vi "EOL Check Sunshade Limits.vi"(7 "Pass? In":bool=TRUE, 8 "Error Table":string[][](array[string]), 9 "Sunshade Close?":bool=TRUE, 10 "Sun Shade Limits":T1 {"Variance" format="%.2g"; "Truncation End" format="%.2g"; "Truncation Start" format="%.2g"; "Avg Max" format="%.2g"; "Avg Min" format="%.2g"; "Overall Max" format="%.2g"; "Overall Min" format="%.2g"}, 11 "Sunshade Calculated Data":dbl[](array[numeric])) -> (0 "Error Table 2":string[][](array[string]), 2 "All Sunshade Data and Limits":dbl[](array[numeric]), 3 "Pass?":bool)   [LabVIEW 2018]
uses:
  05.UserVI's/type defs/17x Sunshade Limts Seq.ctl
panel:
  # "Min"
  # "N"
  # "Min"
  # "Start"
  # "N"
  # "Max"
  # "N"
  # "Max"
  # "N"
  # "End"
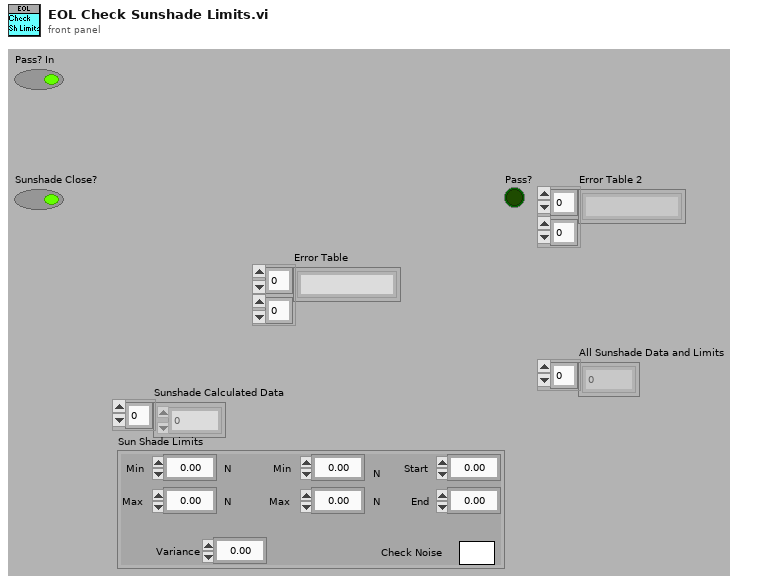
[diagram p1: front panel]
types:
  T1 = typedef "17x Sunshade Limts Seq.ctl" = cluster{"Overall Min":dbl, "Overall Max":dbl, "Avg Min":dbl, "Avg Max":dbl, "Truncation Start":dbl, "Truncation End":dbl, "Variance":dbl, "Check Noise":bool}
  T2 = cluster{"Sunshade Calculated Data":dbl[], "Sun Shade Limits":T1, "Error Table":string[][], "Sunshade Close?":bool, "Pass? In":bool}
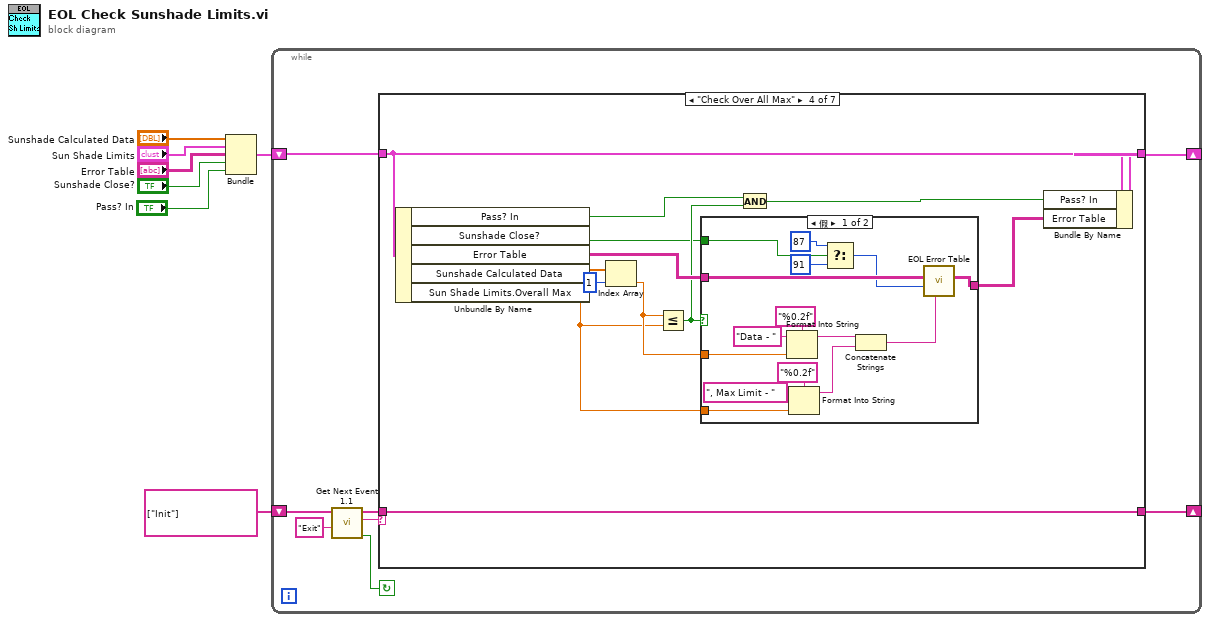
[diagram p0: block diagram]
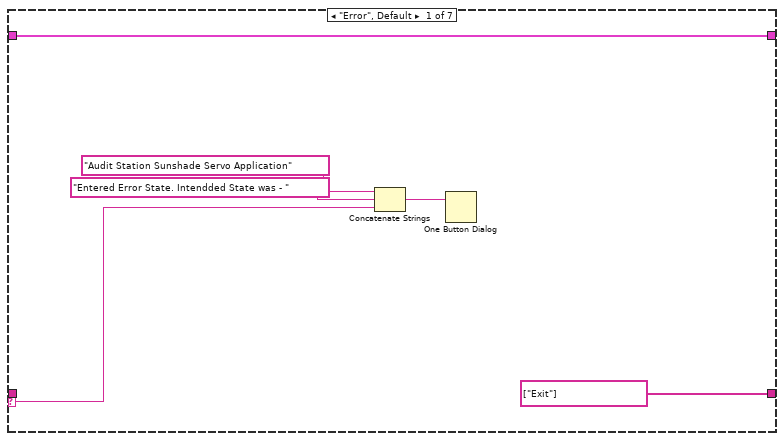
[diagram p2: hidden frame]
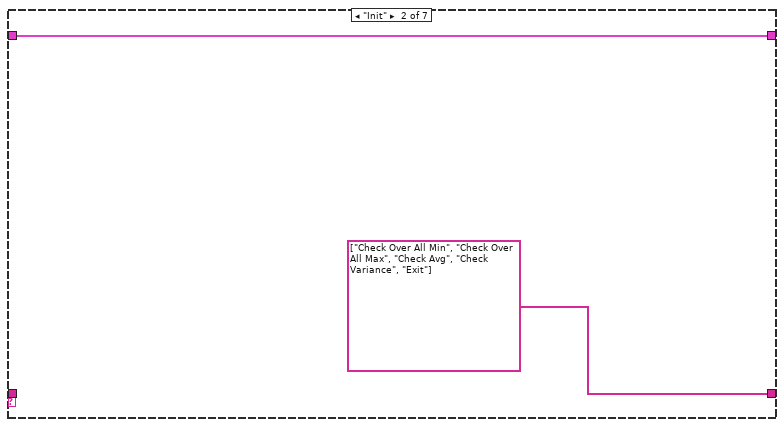
[diagram p3: hidden frame]
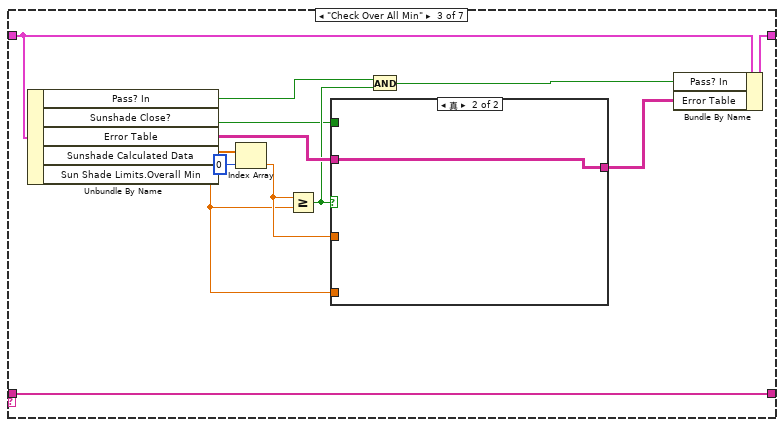
[diagram p4: hidden frame]
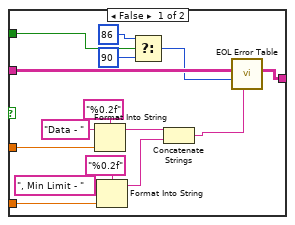
[diagram p5: hidden frame]
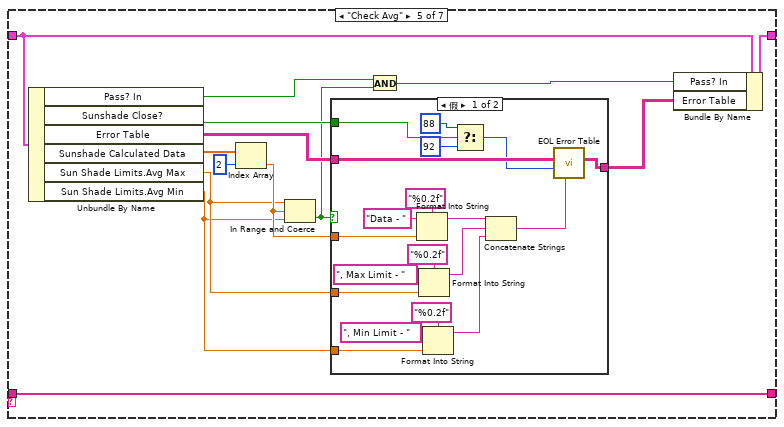
[diagram p7: hidden frame]
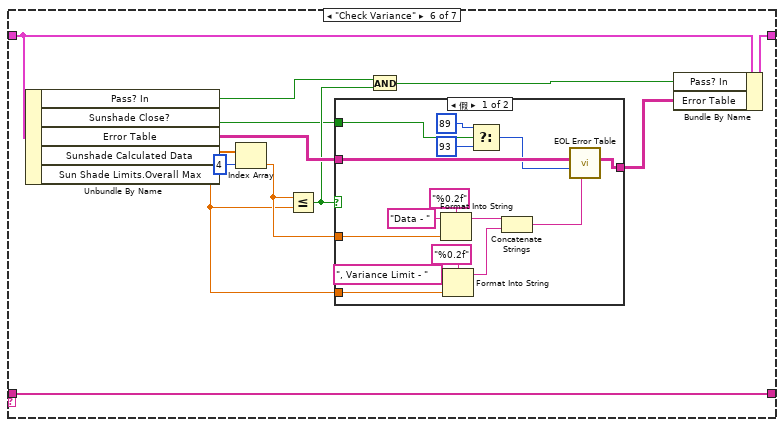
[diagram p9: hidden frame]
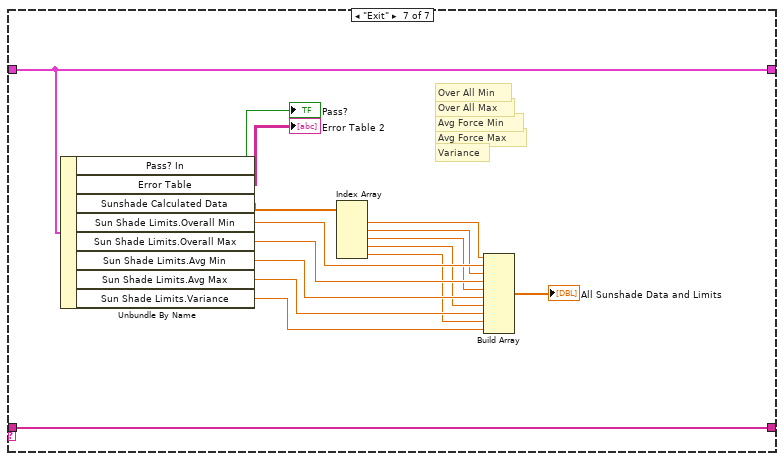
[diagram p11: hidden frame]
diagram:
  n1 = Bundle("Sunshade Calculated Data"="Sunshade Calculated Data", "Sun Shade Limits"="Sun Shade Limits", "Error Table"="Error Table", "Sunshade Close?"="Sunshade Close?", "Pass? In"="Pass? In") -> (w2:T2)  [unwired: 1 in]
  n2 = while {
    shift-right: [w11] -> _
    shift-left: string[] ["Init"] ("event queue out") -> [w10]
    shift-right: [w8] -> _
    shift-left: w2 -> [w9]
    stop <- w14 continue-if-true
    n3 = call "Get Next Event 1.1.vi"("Exit Event"="Exit", "event queue in"=w10) -> ("Condition (Exit:F)"=w14:bool, "next event"=w15:string, "event queue out"=w12:string[])  [unwired: 6 in, 1 out]
    n4 = case shown="\"Check Over All Max\"" w15 {
      selector: w15 -> [w17 _ _ _ _ _ _]
      tunnel: w12 -> [_ _ w29 w58 w89 w121 w160]
      tunnel: [string[] ["Exit"] ("event queue out") string[] ["Check Over All Min", "Check Over All Max", "Check Avg", "Check Variance", "Exit"] ("event queue out") w29 w58 w89 w121 w160] -> w11
      tunnel: w9 -> [w16 w23 w34 w63 w93 w126 w159]
      tunnel: [w16 w23 w30 w59 w90 w122 w159] -> w8
      frame "Error", Default {
        n5 = Concatenate Strings("Audit Station Sunshade Servo Application" ("string"), "Entered Error State. Intendded State was - " ("string"), w17) -> (w20:string)
        n6 = One Button Dialog(message=w20) -> ()  [unwired: 1 in, 1 out]
      }
      frame "Init" {
      }
      frame "Check Over All Min" {
        n7 = Unbundle By Name(w34) -> ("Pass? In"=w33:bool, "Sunshade Close?"=w25:bool, "Error Table"=w35:string[][], "Sunshade Calculated Data"=w36:dbl[], "Sun Shade Limits.Overall Min"=w26:dbl)
        n8 = Index Array(array=w36, index=0) -> (element=w27:dbl)
        n9 = Greater Or Equal?(x=w27, y=w26) -> (x >= y?=w32:bool)
        n10 = case shown="真" w32 {
          tunnel: w35 -> [w51 w52]
          tunnel: w26 -> [w48 _]
          tunnel: [w37 w52] -> w28
          tunnel: w27 -> [w43 _]
          tunnel: w25 -> [w42 _]
          frame False {
            n11 = Format Into String(format string="%0.2f", initial string="Data - ", w43) -> (resulting string=w45:string)  [unwired: 1 in, 1 out]
            n12 = Format Into String(format string="%0.2f", initial string=", Min Limit - ", w48) -> (resulting string=w44:string)  [unwired: 1 in, 1 out]
            n13 = Select(t=u16 86 ("Error No."), s=w42, f=u16 90) -> (s? t:f=w38:u16)
            n14 = Concatenate Strings(w45, w44) -> (w39:string)
            n15 = call "EOL Error Table.vi"("Error Description"=w39, "Error No."=w38, "Error Table In"=w51) -> ("Error Table Out"=w37:string[][])  [unwired: 7 in, 1 out]
          }
          frame True {
          }
        }
        n16 = And(x=w33, y=w32) -> (x .and. y?=w31:bool)
        n17 = Bundle By Name(cluster=w34, "Pass? In"=w31, "Error Table"=w28) -> (w30:T2)
      }
      frame "Check Over All Max" {
        n18 = Unbundle By Name(w63) -> ("Pass? In"=w62:bool, "Sunshade Close?"=w54:bool, "Error Table"=w64:string[][], "Sunshade Calculated Data"=w65:dbl[], "Sun Shade Limits.Overall Max"=w55:dbl)
        n19 = Index Array(array=w65, index=1) -> (element=w56:dbl)
        n20 = Less Or Equal?(x=w56, y=w55) -> (x <= y?=w61:bool)
        n21 = case shown="假" w61 {
          tunnel: w64 -> [w80 w81]
          tunnel: w55 -> [w77 _]
          tunnel: [w66 w81] -> w57
          tunnel: w56 -> [w72 _]
          tunnel: w54 -> [w71 _]
          frame False {
            n22 = Format Into String(format string="%0.2f", initial string="Data - ", w72) -> (resulting string=w74:string)  [unwired: 1 in, 1 out]
            n23 = Format Into String(format string="%0.2f", initial string=", Max Limit - ", w77) -> (resulting string=w73:string)  [unwired: 1 in, 1 out]
            n24 = Select(t=u16 87 ("Error No."), s=w71, f=u16 91) -> (s? t:f=w67:u16)
            n25 = Concatenate Strings(w74, w73) -> (w68:string)
            n26 = call "EOL Error Table.vi"("Error Description"=w68, "Error No."=w67, "Error Table In"=w80) -> ("Error Table Out"=w66:string[][])  [unwired: 7 in, 1 out]
          }
          frame True {
          }
        }
        n27 = And(x=w62, y=w61) -> (x .and. y?=w60:bool)
        n28 = Bundle By Name(cluster=w63, "Pass? In"=w60, "Error Table"=w57) -> (w59:T2)
      }
      frame "Check Avg" {
        n29 = Unbundle By Name(w93) -> ("Pass? In"=w92:bool, "Sunshade Close?"=w87:bool, "Error Table"=w94:string[][], "Sunshade Calculated Data"=w95:dbl[], "Sun Shade Limits.Avg Max"=w84:dbl, "Sun Shade Limits.Avg Min"=w82:dbl)
        n30 = Index Array(array=w95, index=2) -> (element=w85:dbl)
        n31 = In Range and Coerce(upper limit=w84, x=w85, lower limit=w82) -> (In Range?=w83:bool)  [unwired: 1 out]
        n32 = case shown="假" w83 {
          tunnel: w94 -> [w114 w115]
          tunnel: w84 -> [w111 _]
          tunnel: [w96 w115] -> w88
          tunnel: w85 -> [w106 _]
          tunnel: w87 -> [w105 _]
          tunnel: w82 -> [w100 _]
          frame False {
            n33 = Format Into String(format string="%0.2f", initial string="Data - ", w106) -> (resulting string=w108:string)  [unwired: 1 in, 1 out]
            n34 = Format Into String(format string="%0.2f", initial string=", Max Limit - ", w111) -> (resulting string=w107:string)  [unwired: 1 in, 1 out]
            n35 = Format Into String(format string="%0.2f", initial string=", Min Limit - ", w100) -> (resulting string=w99:string)  [unwired: 1 in, 1 out]
            n36 = Select(t=u16 88 ("Error No."), s=w105, f=u16 92) -> (s? t:f=w97:u16)
            n37 = Concatenate Strings(w108, w107, w99) -> (w98:string)
            n38 = call "EOL Error Table.vi"("Error Description"=w98, "Error No."=w97, "Error Table In"=w114) -> ("Error Table Out"=w96:string[][])  [unwired: 7 in, 1 out]
          }
          frame True {
          }
        }
        n39 = And(x=w92, y=w83) -> (x .and. y?=w91:bool)
        n40 = Bundle By Name(cluster=w93, "Pass? In"=w91, "Error Table"=w88) -> (w90:T2)
      }
      frame "Check Variance" {
        n41 = Unbundle By Name(w126) -> ("Pass? In"=w125:bool, "Sunshade Close?"=w117:bool, "Error Table"=w127:string[][], "Sunshade Calculated Data"=w128:dbl[], "Sun Shade Limits.Overall Max"=w118:dbl)
        n42 = Index Array(array=w128, index=4) -> (element=w119:dbl)
        n43 = Less Or Equal?(x=w119, y=w118) -> (x <= y?=w124:bool)
        n44 = case shown="假" w124 {
          tunnel: w127 -> [w143 w144]
          tunnel: w118 -> [w140 _]
          tunnel: [w129 w144] -> w120
          tunnel: w119 -> [w135 _]
          tunnel: w117 -> [w134 _]
          frame False {
            n45 = Format Into String(format string="%0.2f", initial string="Data - ", w135) -> (resulting string=w137:string)  [unwired: 1 in, 1 out]
            n46 = Format Into String(format string="%0.2f", initial string=", Variance Limit - ", w140) -> (resulting string=w136:string)  [unwired: 1 in, 1 out]
            n47 = Select(t=u16 89 ("Error No."), s=w134, f=u16 93) -> (s? t:f=w130:u16)
            n48 = Concatenate Strings(w137, w136) -> (w131:string)
            n49 = call "EOL Error Table.vi"("Error Description"=w131, "Error No."=w130, "Error Table In"=w143) -> ("Error Table Out"=w129:string[][])  [unwired: 7 in, 1 out]
          }
          frame True {
          }
        }
        n50 = And(x=w125, y=w124) -> (x .and. y?=w123:bool)
        n51 = Bundle By Name(cluster=w126, "Pass? In"=w123, "Error Table"=w120) -> (w122:T2)
      }
      frame "Exit" {
        # "Variance"
        # "Avg Force Max"
        # "Avg Force Min"
        # "Over All Max"
        # "Over All Min"
        n52 = Unbundle By Name(w159) -> ("Pass? In"=→"Pass?":bool, "Error Table"=→"Error Table 2":string[][], "Sunshade Calculated Data"=w156:dbl[], "Sun Shade Limits.Overall Min"=w154:dbl, "Sun Shade Limits.Overall Max"=w152:dbl, "Sun Shade Limits.Avg Min"=w150:dbl, "Sun Shade Limits.Avg Max"=w148:dbl, "Sun Shade Limits.Variance"=w146:dbl)
        n53 = Index Array(array=w156) -> (element #1=w155:dbl, element #2=w153:dbl, element #3=w151:dbl, element #4=w149:dbl, element #5=w147:dbl)  [unwired: 5 in]
        n54 = Build Array(w155, w154, w153, w152, w151, w150, w149, w148, w147, w146) -> (→"All Sunshade Data and Limits":dbl[])
      }
    }
  }
